vi "Set Configuration Error.vi"(4 "Is Error? (T)":bool=TRUE, 6 "Message":string, 8 "error in (no error)":errorcluster, 9 "NationalInstruments.VeriStand.ErrorCode":i32(ring) items=["Success"=0, "NoProjectOpen"=-307992, "SequenceCompileError"=-307988, "SessionAlreadyDeployed"=-307984, "SessionNotDeployed"=-307982, "SequenceNotFoundInSession"=-307981, "StimulusProfileSessionLocked"=-307980, "EmptyNodeName"=-307930, "NodeAlreadyExistsByName"=-307926, "NumberOfCoefficientsOutOfRange"=-307884, "DownloadFileError"=-307872, "IncorrectLogFileName"=-307871, "LogTriggerConditionSyntaxError"=-307868, "DuplicateLogSessionName"=-307867, "LogSessionNotFound"=-307865, "ChannelLengthMismatch"=-307830, "NodeNotFoundDuringCompile"=-307829, "ChannelNodeRemoved"=-307828, "NotAChannel"=-307825, "NotAWaveform"=-307824, "STIFileError"=-307784, "DependenciesCycle"=-307783, "ChannelNotFoundInLogFile"=-307782, "ChannelGroupNotFoundInLogFile"=-307781, "GatewayNotOnLocalhost"=-307780, "NotEnoughDynamicDataSharingSpace"=-307738, "TargetMissingDataSharingDevice"=-307737, "ChannelMappingsSizeMismatch"=-307728, "DuplicateChannelAliasMappings"=-307711, "NotAnInlineCustomDevice"=-307710, "IncompatibleModel"=-307703, "ModelDimensionMismatch"=-307702, "SLSCChassisLoadFailed"=-307691, "TargetDisabled"=-307689, "MismatchedLengths"=-307687, "TargetInvalid"=-307686, "ParameterNotFound"=-307685, "ServerPortAlreadyInUse"=-307684, "TargetDisconnected"=-307682, "ServiceConfigurationFile"=-307681, "ModelParameterFileParseError"=-307680, "NoActionRequired"=-307677, "InputParameterInvalid"=-307676, "HostRunningDifferentSystemDefinition"=-307671, "ChannelNotScalable"=-307668, "ChannelCannotBeFaulted"=-307666, "ChannelNotWritable"=-307665, "ChannelNotReadable"=-307664, "Timeout"=-307663, "NodeNotFound"=-307662, "SystemDefinitionDeploymentFailure"=-307661, "SystemDefinitionDeploymentTimeout"=-307660, "EmptyPassword"=-307659, "SystemDefinitionAlreadyActive"=-307658, "InvalidConfigurationPassword"=-307657, "NoSystemDefinitionLoaded"=-307656, "ComponentNotAvailable"=-307655, "NotDeployed"=-307654, "InvalidFile"=-307653, "FailedServerConnection"=-307652, "FunctionNotSupported"=-307651, "UnexpectedError"=-307650, "UnmappedAlias"=-307617, "InvalidStreamConditionForDataType"=-307554, "WaveformDataTypeMismatch"=-307553, "InvalidDaqPluginFile"=-307526, "FileVersionUnsupported"=-307525], 10 "Key":string, 11 "Item Ref in":T1 format="%.0x") -> (0 "error out":errorcluster, 3 "Item Ref out":T1 format="%.0x")   [LabVIEW 2019, in "Routing and Faulting System Explorer.lvlib"]
uses:
  Routing and Faulting System Explorer.lvlib
  <vilib>/NI/NI VeriStand Error API/VeriStand Error API.lvlib
  <vilib>/NI/NI VeriStand Error API/VeriStand Error.ctl
  <vilib>/NI VeriStand/Custom Device API/Custom Device Item Ref.ctl
  <vilib>/NI VeriStand/Custom Device API/Custom Device API.lvlib
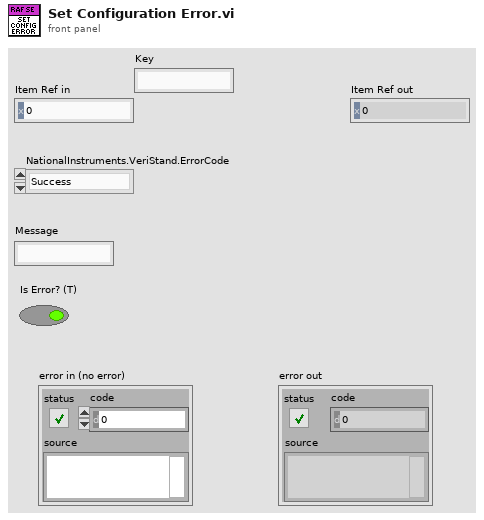
[diagram p1: front panel]
types:
  T1 = typedef "Custom Device API.lvlib/Custom Device Item Ref.ctl" = u64
  T2 = typedef "VeriStand Error API.lvlib/VeriStand Error.ctl" = cluster{"status":bool, "code":i32, "message":string}
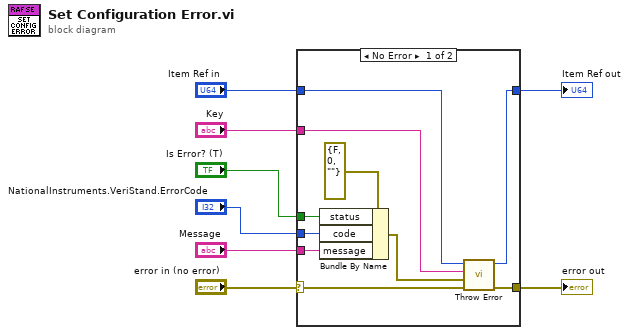
[diagram p0: block diagram]
diagram:
  n1 = case shown="No Error" "error in (no error)" {
    selector: "error in (no error)" -> [w11 w19]
    tunnel: "Is Error? (T)" -> [w17 _]
    tunnel: "NationalInstruments.VeriStand.ErrorCode" -> [w16 _]
    tunnel: "Message" -> [w15 _]
    tunnel: "Item Ref in" -> [w13 w20]
    tunnel: "Key" -> [w12 _]
    tunnel: [w10 w19] -> w2
    tunnel: [w9 w20] -> w1
    frame No Error {
      n2 = Bundle By Name(cluster=T2 {"status"=FALSE, "code"=0, "message"=""} ("VeriStand Error In"), "status"=w17, "code"=w16, "message"=w15) -> (w14:T2)
      n3 = call <vilib>:"Throw Error.vi"("error in"=w11, "VeriStand Error In"=w14, "Key"=w12, "Item Ref in"=w13) -> ("error out"=w10:errorcluster, "Item Ref out"=w9:T1)  [unwired: 6 in]
    }
    frame Error {
    }
  }
  "Item Ref out" <- w1
  "error out" <- w2
